vi "Query with Scalar 64bit Integer Result.vi"(8 "error in (no error)":errorcluster, 10 "Query string":string, 11 "mysql in":refnum<class "mysql.lvclass">) -> (0 "error out":errorcluster, 2 "Result":i64, 3 "mysql out":refnum<class "mysql.lvclass">)   [LabVIEW 2020, in "mysql.lvlib" / "mysql.lvclass"]
uses:
  mysql.lvclass
  2befb942-14e7-4967-aaa5-f6be69aca6b8.vi
  2befb942-14e7-4967-aaa5-f6be69aca6b8.vi/806c8009-165f-4631-8400-09e9b69867cc.vi
  private/Mysql command.vi
  private/Mysql data reader Scalar I64.vi
  private/ping connection and reopen if needed.vi
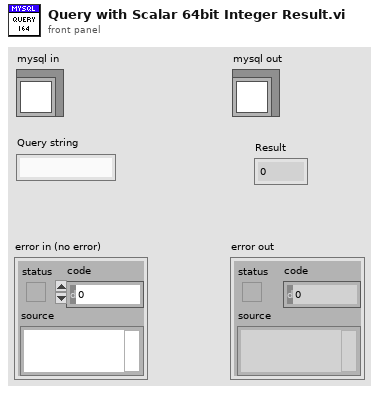
[diagram p1: front panel]
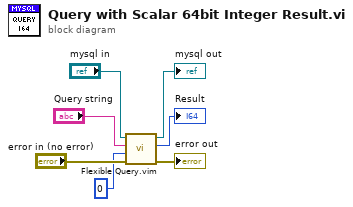
[diagram p0: block diagram]
diagram:
  n1 = call "Flexible Query.vim"("error in (no error)"="error in (no error)", "Type in"=i64 0 ("Result 2"), "Query string"="Query string", "mysql in"="mysql in") -> ("error out"=→"error out":errorcluster, "Result"=→"Result":i64, "mysql out"=→"mysql out":refnum<class "mysql.lvclass">)  [unwired: 5 in]
